vi "Custom errors handler-Acq.vi"(9 "Imaging Protocol":T1, 11 "code":i32) -> ()   [LabVIEW 2017]
uses:
  Typedefs/Imaging Protocols enum.ctl
  Typedefs/Top level VI states.ctl
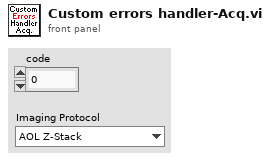
[diagram p1: front panel]
types:
  T1 = typedef "Imaging Protocols enum.ctl" = enum16{"AOL Z-Stack", "Motor Z Stack", "Functional Acquisition", "Single Plane Acquisition", "Volume Acquisition", "Live Imaging", "Live Plane Imaging", "Live Volume Imaging"}
  T2 = typedef "Top level VI states.ctl" = enum16{"None", "Initialise UI", "<STACK PROTOCOL STATES>", "AOL Zstack-START", "AOL Zstack-STOP", "Motor Zstack-START", "Motor Zstack-STOP", "<ACQUISITION PROTOCOL STATES> ", "Functional Acquisition-START", "Functional Acquisition-STOP", "Single Plane Acquisition-START", "Single Plane Acquisition-STOP", "Volume Acquisition-START", "Volume Acquisition-STOP", "<LIVE IMAGING PROTOCOL STATES>", "Live Imaging-START", "Live Imaging-STOP", "Live Plane Imaging-START", "Live Plane Imaging-STOP", "Live Volume Imaging-START", "Live Volume Imaging-STOP", "<MOVEMENT CORRECTION PROTOCOL STATES>", "Background MovCor-START", "Background MovCor-STOP", "EXIT"}
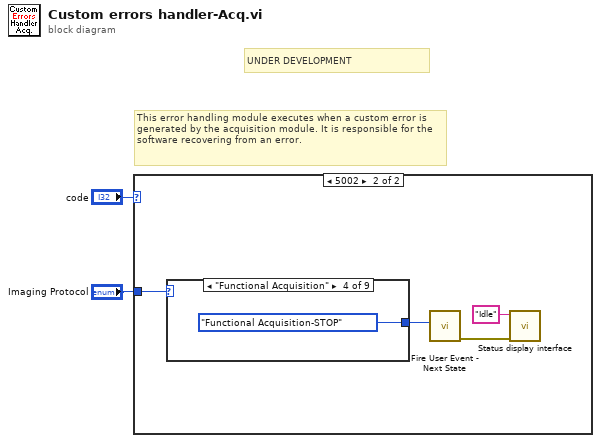
[diagram p0: block diagram]
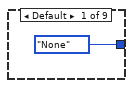
[diagram p3: hidden frame]
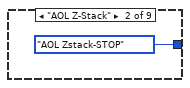
[diagram p4: hidden frame]
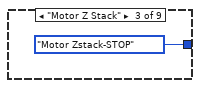
[diagram p5: hidden frame]
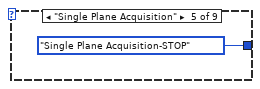
[diagram p6: hidden frame]
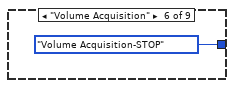
[diagram p7: hidden frame]
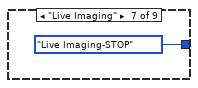
[diagram p8: hidden frame]
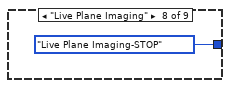
[diagram p9: hidden frame]
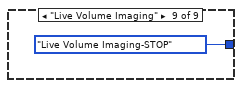
[diagram p10: hidden frame]
diagram:
  # "UNDER DEVELOPMENT"
  # "This error handling module executes when a custom error is generated by the acquisition module. It is responsible for the software recovering from an error."
  n1 = case shown="5002" "code" {
    tunnel: "Imaging Protocol" -> [_ w6]
    frame 0, Default {
    }
    frame 5002 {
      n2 = case shown="\"Functional Acquisition\"" w6 {
        tunnel: [Top_level_VI_states."None" ("State") Top_level_VI_states."AOL Zstack-STOP" ("State") Top_level_VI_states."Motor Zstack-STOP" ("State") Top_level_VI_states."Functional Acquisition-STOP" ("State") Top_level_VI_states."Single Plane Acquisition-STOP" ("State") Top_level_VI_states."Volume Acquisition-STOP" ("State") Top_level_VI_states."Live Imaging-STOP" ("State") Top_level_VI_states."Live Plane Imaging-STOP" ("State") Top_level_VI_states."Live Volume Imaging-STOP" ("State")] -> w4
        frame Default {
        }
        frame "AOL Z-Stack" {
        }
        frame "Motor Z Stack" {
        }
        frame "Functional Acquisition" {
        }
        frame "Single Plane Acquisition" {
        }
        frame "Volume Acquisition" {
        }
        frame "Live Imaging" {
        }
        frame "Live Plane Imaging" {
        }
        frame "Live Volume Imaging" {
        }
      }
      n3 = call "Fire User Event - Next State.vi"("\"UI Handler loop\" case to execute"=w4) -> ("Error Out"=w3:errorcluster)  [unwired: 10 in]
      n4 = call "Status display interface.vi"("error in (no error)"=w3, "Message"="Idle") -> ()  [unwired: 9 in, 1 out]
    }
  }
